vi "NanoStageGetPositions.vi"(7 "error in (no error)":errorcluster, 10 "Config In":T1) -> (0 "error out":errorcluster, 2 "Positions":cluster{"Time":dbl, "x":dbl, "y":dbl, "z":dbl}, 3 "Config Out":T1)   [LabVIEW 2019]
doc: "Generates sample waveforms according to the signal type in the HW Config input."
uses:
  Settings/Settings.ctl
  Support/Hardware Configuration.ctl
  Support/Camera Configuration.ctl
  E:/DevHardSoftware/MMicroscopy/HardwareAdapter/Camera/Dependencies/PVCamNET.dll
  Camera/Dependencies/PVCamNET.dll
  <vilib>/userdefined/High Color/IMAQdx.ctl
  E:/DevHardSoftware/MMicroscopy/HardwareAdapter/Lasers/Dependencies/Oxxius_Boxx.dll
  Lasers/Dependencies/Oxxius_Boxx.dll
  Logging/Logging Configuration.ctl
  controls/UI Configuration.ctl
  <vilib>/numeric/Random Number (Range) U64.vi
  <vilib>/numeric/sub_Random U32.vi
  Dependencies/Madlib.dll
  Logging/Logging.lvlib
  Settings/Settings.lvlib
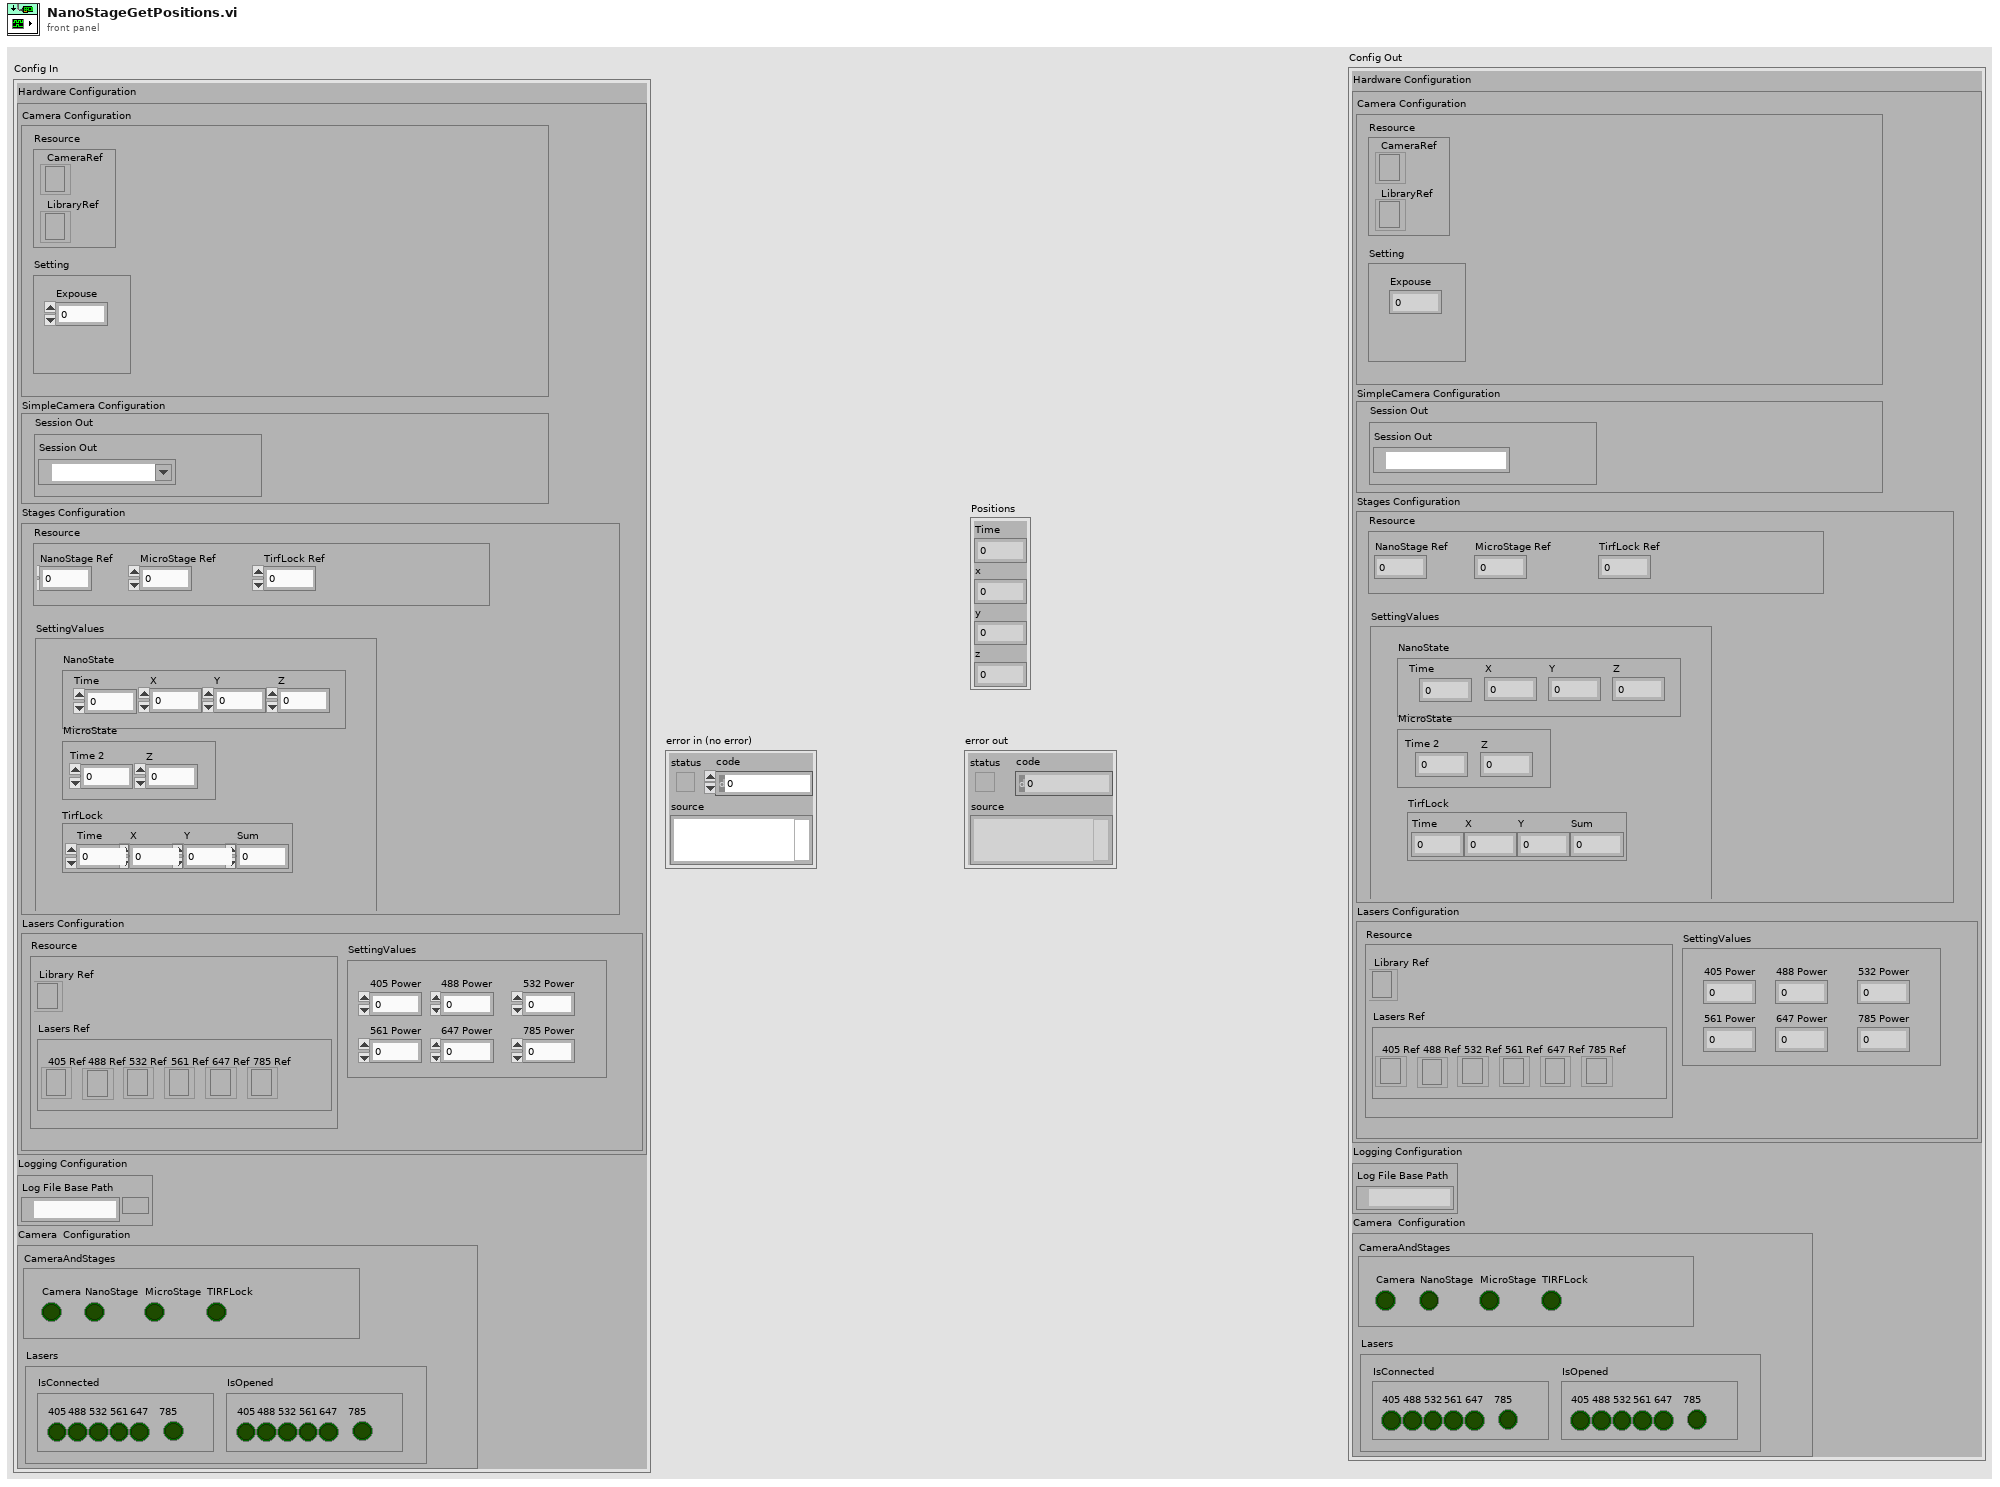
[diagram p1: front panel]
types:
  T1 = typedef "Settings.lvlib/Settings.ctl" = cluster{"Hardware Configuration":T2, "Logging Configuration":T5, "HardWare Status":cluster{"CameraAndStages":T6, "Lasers":cluster{"IsConnected":cluster{"405":bool, "488":bool, "532":bool, "561":bool, "647":bool, "785":bool}, "IsOpened":cluster{"405":bool, "488":bool, "532":bool, "561":bool, "647":bool, "785":bool}}}}
  T2 = typedef "Hardware Configuration.ctl" = cluster{"Camera Configuration":T3, "SimpleCamera Configuration":cluster{"Resource":cluster{"Session Out":T4}}, "Stages Configuration":cluster{"Resource":cluster{"NanoStage Ref":i32, "MicroStage Ref":i32, "TirfLock Ref":i32}, "SettingValues":cluster{"NanoState":cluster{"Time":dbl, "X":dbl, "Y":dbl, "Z":dbl}, "MicroState":cluster{"Time 2":dbl, "Z":dbl}, "TirfLock":cluster{"Time":dbl, "X":dbl, "Y":dbl, "Sum":dbl}}}, "Lasers Configuration":cluster{"SettingValues":cluster{"405 Power":i32, "488 Power":i32, "532 Power":i32, "561 Power":i32, "647 Power":i32, "785 Power":i32}, "Resource":cluster{"Library Ref":refnum<k24>, "Lasers Ref":cluster{"405 Ref":refnum<k24>, "488 Ref":refnum<k24>, "532 Ref":refnum<k24>, "561 Ref":refnum<k24>, "647 Ref":refnum<k24>, "785 Ref":refnum<k24>}}}}
  T3 = typedef "Camera Configuration.ctl" = cluster{"Resource":cluster{"CameraRef":refnum<k24>, "LibraryRef":refnum<k24>}, "Setting":cluster{"Expouse":dbl}}
  T4 = typedef "IMAQdx.ctl" = refnum<k21>
  T5 = typedef "Logging.lvlib/Logging Configuration.ctl" = cluster{"Log File Base Path":path}
  T6 = typedef "UI Configuration.ctl" = cluster{"Camera":bool, "NanoStage":bool, "MicroStage":bool, "TIRFLock":bool}
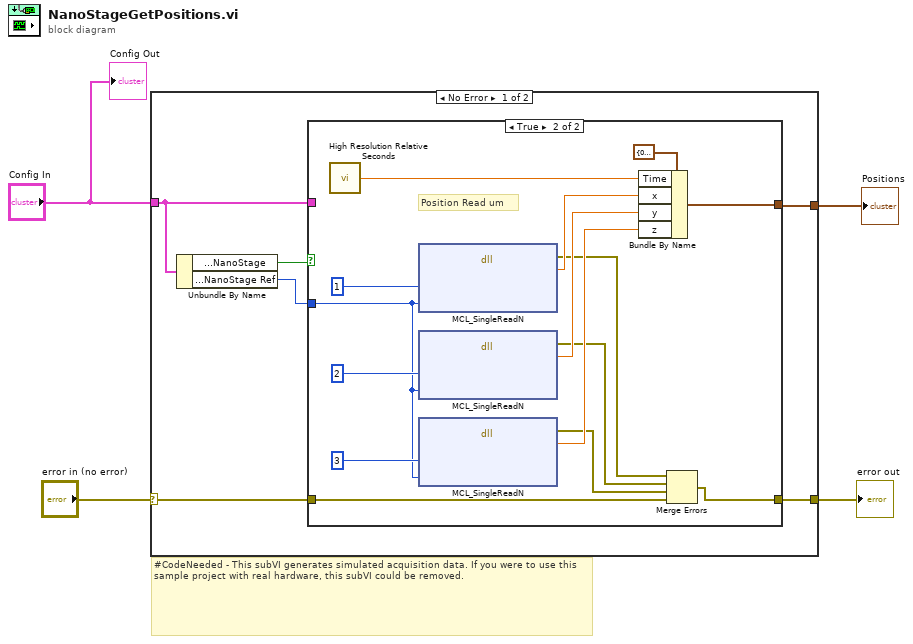
[diagram p0: block diagram]
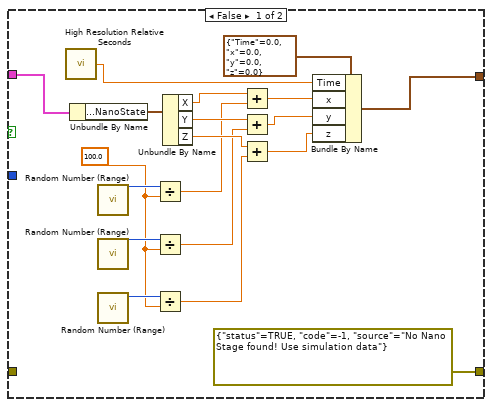
[diagram p2: hidden frame]
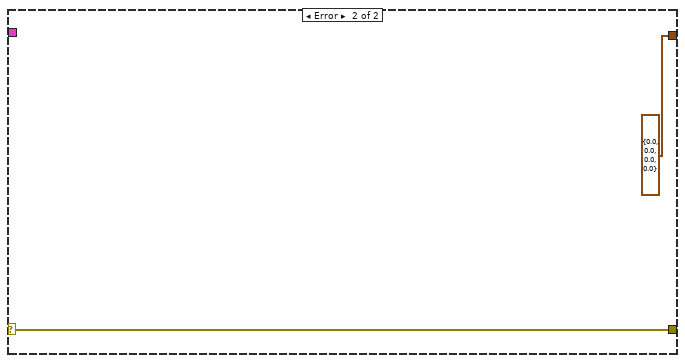
[diagram p3: hidden frame]
diagram:
  # "#CodeNeeded - This subVI generates simulated acquisition data. If you were to use this sample project with real hardware, this subVI could be removed."
  n1 = case shown="No Error" "error in (no error)" {
    selector: "error in (no error)" -> [w6 w45]
    tunnel: [w7 w45] -> w3
    tunnel: "Config In" -> [w5 _]
    tunnel: [w10 cluster{"Time":dbl, "x":dbl, "y":dbl, "z":dbl} {"Time"=0.0, "x"=0.0, "y"=0.0, "z"=0.0} ("RawImage")] -> w1
    frame No Error {
      n2 = Unbundle By Name(w5) -> ("HardWare Status.CameraAndStages.NanoStage"=w9:bool, "Hardware Configuration.Stages Configuration.Resource.NanoStage Ref"=w8:i32)
      n3 = case shown="True" w9 {
        tunnel: [w27 w44] -> w10
        tunnel: w8 -> [_ w38]
        tunnel: [errorcluster {"status"=TRUE, "code"=-1, "source"="No Nano Stage found! Use simulation data"} ("error IO") w33] -> w7
        tunnel: w6 -> [_ w34]
        tunnel: w5 -> [w25 _]
        frame False {
          w14 = 100.0 ("Time")
          n4 = call <vilib>:"High Resolution Relative Seconds.vi"() -> ("relative seconds"=w26:dbl)
          n5 = Unbundle By Name(w25) -> ("Hardware Configuration.Stages Configuration.SettingValues.NanoState"=w24:cluster{"Time":dbl, "X":dbl, "Y":dbl, "Z":dbl})
          n6 = call-poly <vilib>:"Random Number (Range).vi"() -> ("number"=w23:u64)  [unwired: 11 in]
          n7 = call-poly <vilib>:"Random Number (Range).vi"() -> ("number"=w21:u64)  [unwired: 11 in]
          n8 = call-poly <vilib>:"Random Number (Range).vi"() -> ("number"=w22:u64)  [unwired: 11 in]
          n9 = Divide(x=w23, y=w14) -> (x/y=w15:dbl)
          n10 = Divide(x=w21, y=w14) -> (x/y=w16:dbl)
          n11 = Divide(x=w22, y=w14) -> (x/y=w17:dbl)
          n12 = Unbundle By Name(w24) -> ("X"=w20:dbl, "Y"=w19:dbl, "Z"=w18:dbl)
          n13 = Add(x=w20, y=w15) -> (x+y=w13:dbl)
          n14 = Add(x=w19, y=w16) -> (x+y=w12:dbl)
          n15 = Add(x=w18, y=w17) -> (x+y=w11:dbl)
          n16 = Bundle By Name(cluster=cluster{"Time":dbl, "x":dbl, "y":dbl, "z":dbl} {"Time"=0.0, "x"=0.0, "y"=0.0, "z"=0.0} ("NanoStage"), "Time"=w26, "x"=w13, "y"=w12, "z"=w11) -> (w27:cluster{"Time":dbl, "x":dbl, "y":dbl, "z":dbl})
        }
        frame True {
          # "Position Read um"
          n17 = call <vilib>:"High Resolution Relative Seconds.vi"() -> ("relative seconds"=w40:dbl)
          n18 = dll-call lib="E:/DevHardSoftware/MMicroscopy/HardwareAdapter/Stages/Dependencies/Madlib.dll" fn="MCL_SingleReadN"("axis"=u32 1, "handle"=w38) -> (error out=w30:errorcluster, w37:dbl)  [unwired: 5 in, 1 out]
          n19 = dll-call lib="E:/DevHardSoftware/MMicroscopy/HardwareAdapter/Stages/Dependencies/Madlib.dll" fn="MCL_SingleReadN"("axis"=u32 2, "handle"=w38) -> (error out=w31:errorcluster, w36:dbl)  [unwired: 5 in, 1 out]
          n20 = dll-call lib="E:/DevHardSoftware/MMicroscopy/HardwareAdapter/Stages/Dependencies/Madlib.dll" fn="MCL_SingleReadN"("axis"=u32 3, "handle"=w38) -> (error out=w32:errorcluster, w35:dbl)  [unwired: 5 in, 1 out]
          n21 = Bundle By Name(cluster=cluster{"Time":dbl, "x":dbl, "y":dbl, "z":dbl} {"Time"=0.0, "x"=0.0, "y"=0.0, "z"=0.0} ("RawImage"), "Time"=w40, "x"=w37, "y"=w36, "z"=w35) -> (w44:cluster{"Time":dbl, "x":dbl, "y":dbl, "z":dbl})
          n22 = Merge Errors(w30, w31, w32, w34) -> (w33:errorcluster)
        }
      }
    }
    frame Error {
    }
  }
  "error out" <- w3
  "Positions" <- w1
  "Config Out" <- "Config In"
